vi "XGT 연속읽기 (독립)ONOFF.vi"() -> (1 "배열":i32[](array[numeric]))   [LabVIEW 2012]
uses:
  <vilib>/Instr/_visa.llb/VISA Configure Serial Port (Instr).vi
panel:
  in  "length":i32=6
  out "데이터 개수":string
  out "에러 코드":string
  out "Waveform Graph":i32[](graph)
  out "Array":i32[](array[numeric])
  out "Serial Settings:Number of Bytes at Serial Port":u32
  in  "stop bits (10: 1 bit)":u16(ring)=10 caption="정지 비트(10: 1비트)" items=["1.0"=10, "1.5"=15, "2.0"=20]
  in  "parity (0:none)":enum16{"None", "Odd", "Even", "Mark", "Space"}(ring) caption="패리티(0:없음)"
  in  "data bits (8)":u16=8 caption="데이터 비트(8)" min=5 max=8 step=1
  in  "baud rate (9600)":u32=9600 caption="보 전송속도(9600)"
  in  "VISA resource name":refnum<visa-resource-name>="COM4" caption="VISA 리소스 이름"
  # "응답"
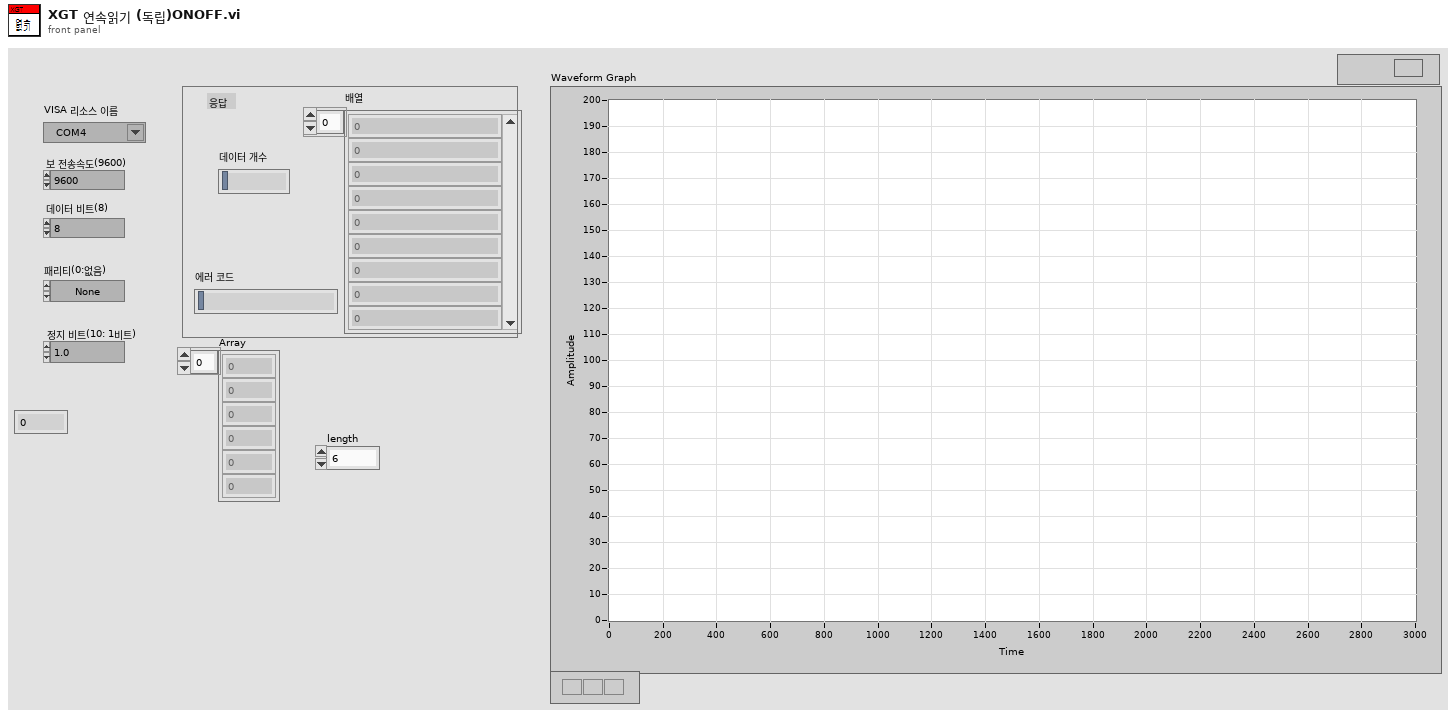
[diagram p1: front panel]
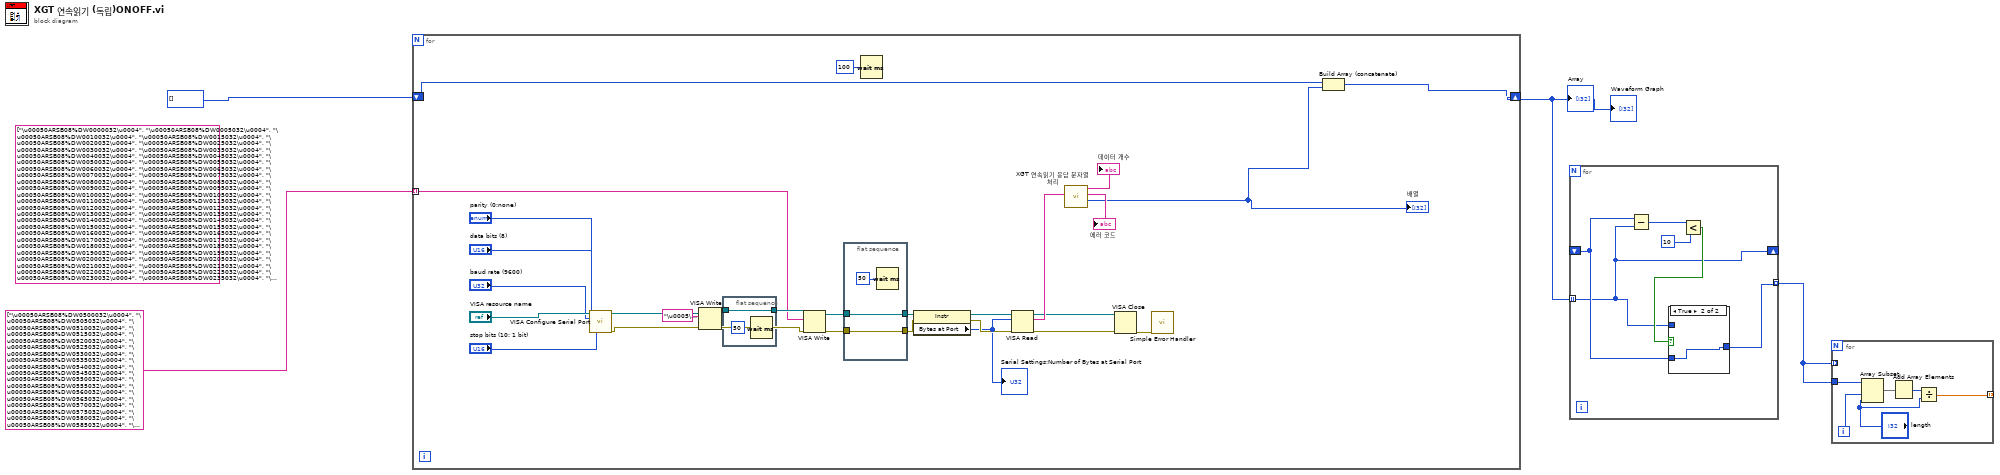
[diagram p0: block diagram]
diagram:
  (unwired) string[] ["\u00050ARSB08%DW0000032\u0004", "\u00050ARSB08%DW0005032\u0004", "\u00050ARSB08%DW0010032\u0004", "\u00050ARSB08%DW0015032\u0004", "\u00050ARSB08%DW0020032\u0004", "\u00050ARSB08%DW0025032\u0004", "\u00050ARSB08%DW0030032\u0004", "\u00050ARSB08%DW0035032\u0004", "\u00050ARSB08%DW0040032\u0004", "\u00050ARSB08%DW0045032\u0004", "\u00050ARSB08%DW0050032\u0004", "\u00050ARSB08%DW0055032\u0004", "\u00050ARSB08%DW0060032\u0004", "\u00050ARSB08%DW0065032\u0004", "\u00050ARSB08%DW0070032\u0004", "\u00050ARSB08%DW0075032\u0004", "\u00050ARSB08%DW0080032\u0004", "\u00050ARSB08%DW0085032\u0004", "\u00050ARSB08%DW0090032\u0004", "\u00050ARSB08%DW0095032\u0004", "\u00050ARSB08%DW0100032\u0004", "\u00050ARSB08%DW0105032\u0004", "\u00050ARSB08%DW0110032\u0004", "\u00050ARSB08%DW0115032\u0004", "\u00050ARSB08%DW0120032\u0004", "\u00050ARSB08%DW0125032\u0004", "\u00050ARSB08%DW0130032\u0004", "\u00050ARSB08%DW0135032\u0004", "\u00050ARSB08%DW0140032\u0004", "\u00050ARSB08%DW0145032\u0004", "\u00050ARSB08%DW0150032\u0004", "\u00050ARSB08%DW0155032\u0004", "\u00050ARSB08%DW0160032\u0004", "\u00050ARSB08%DW0165032\u0004", "\u00050ARSB08%DW0170032\u0004", "\u00050ARSB08%DW0175032\u0004", "\u00050ARSB08%DW0180032\u0004", "\u00050ARSB08%DW0185032\u0004", "\u00050ARSB08%DW0190032\u0004", "\u00050ARSB08%DW0195032\u0004", "\u00050ARSB08%DW0200032\u0004", "\u00050ARSB08%DW0205032\u0004", "\u00050ARSB08%DW0210032\u0004", "\u00050ARSB08%DW0215032\u0004", "\u00050ARSB08%DW0220032\u0004", "\u00050ARSB08%DW0225032\u0004", "\u00050ARSB08%DW0230032\u0004", "\u00050ARSB08%DW0235032\u0004", "\u00050ARSB08%DW0240032\u0004", "\u00050ARSB08%DW0245032\u0004", "\u00050ARSB08%DW0250032\u0004", "\u00050ARSB08%DW0255032\u0004", "\u00050ARSB08%DW0260032\u0004", "\u00050ARSB08%DW0265032\u0004", "\u00050ARSB08%DW0270032\u0004", "\u00050ARSB08%DW0275032\u0004", "\u00050ARSB08%DW0280032\u0004", "\u00050ARSB08%DW0285032\u0004", "\u00050ARSB08%DW0290032\u0004", "\u00050ARSB08%DW0295032\u0004"] ("Array")
  n1 = for {
    tunnel: string[] ["\u00050ARSB08%DW0500032\u0004", "\u00050ARSB08%DW0505032\u0004", "\u00050ARSB08%DW0510032\u0004", "\u00050ARSB08%DW0515032\u0004", "\u00050ARSB08%DW0520032\u0004", "\u00050ARSB08%DW0525032\u0004", "\u00050ARSB08%DW0530032\u0004", "\u00050ARSB08%DW0535032\u0004", "\u00050ARSB08%DW0540032\u0004", "\u00050ARSB08%DW0545032\u0004", "\u00050ARSB08%DW0550032\u0004", "\u00050ARSB08%DW0555032\u0004", "\u00050ARSB08%DW0560032\u0004", "\u00050ARSB08%DW0565032\u0004", "\u00050ARSB08%DW0570032\u0004", "\u00050ARSB08%DW0575032\u0004", "\u00050ARSB08%DW0580032\u0004", "\u00050ARSB08%DW0585032\u0004", "\u00050ARSB08%DW0590032\u0004", "\u00050ARSB08%DW0595032\u0004", "\u00050ARSB08%DW0600032\u0004", "\u00050ARSB08%DW0605032\u0004", "\u00050ARSB08%DW0610032\u0004", "\u00050ARSB08%DW0615032\u0004", "\u00050ARSB08%DW0620032\u0004", "\u00050ARSB08%DW0625032\u0004", "\u00050ARSB08%DW0630032\u0004", "\u00050ARSB08%DW0635032\u0004", "\u00050ARSB08%DW0640032\u0004", "\u00050ARSB08%DW0645032\u0004", "\u00050ARSB08%DW0650032\u0004", "\u00050ARSB08%DW0655032\u0004", "\u00050ARSB08%DW0660032\u0004", "\u00050ARSB08%DW0665032\u0004", "\u00050ARSB08%DW0670032\u0004", "\u00050ARSB08%DW0675032\u0004", "\u00050ARSB08%DW0680032\u0004", "\u00050ARSB08%DW0685032\u0004", "\u00050ARSB08%DW0690032\u0004", "\u00050ARSB08%DW0695032\u0004", "\u00050ARSB08%DW0700032\u0004", "\u00050ARSB08%DW0705032\u0004", "\u00050ARSB08%DW0710032\u0004", "\u00050ARSB08%DW0715032\u0004", "\u00050ARSB08%DW0720032\u0004", "\u00050ARSB08%DW0725032\u0004", "\u00050ARSB08%DW0730032\u0004", "\u00050ARSB08%DW0735032\u0004", "\u00050ARSB08%DW0740032\u0004", "\u00050ARSB08%DW0745032\u0004", "\u00050ARSB08%DW0750032\u0004", "\u00050ARSB08%DW0755032\u0004", "\u00050ARSB08%DW0760032\u0004", "\u00050ARSB08%DW0765032\u0004", "\u00050ARSB08%DW0770032\u0004", "\u00050ARSB08%DW0775032\u0004", "\u00050ARSB08%DW0780032\u0004", "\u00050ARSB08%DW0785032\u0004", "\u00050ARSB08%DW0790032\u0004", "\u00050ARSB08%DW0795032\u0004"] ("Array") -> [w8] mode=indexing
    shift-right: [w6] -> w1
    shift-left: i32[] [] -> [w5]
    n2 = call-poly "VISA Configure Serial Port"("VISA resource name"="VISA resource name", "baud rate (9600)"="baud rate (9600)", "data bits (8)"="data bits (8)", "parity (0:none)"="parity (0:none)", "stop bits (10: 1 bit)"="stop bits (10: 1 bit)") -> ("VISA resource name out"=w17:refnum<visa-resource-name>, "error out"=w16:errorcluster)  [unwired: 9 in]
    n3 = VISA Write(VISA resource name=w17, write buffer="\u0005\u0004", error in (no error)=w16) -> (VISA resource name out=w14:refnum<visa-resource-name>, error out=w15:errorcluster)  [unwired: 1 out]
    n4 = flat-sequence {
      tunnel: w14 -> [w35]
      tunnel: [w35] -> w13
      frame #0 {
        n5 = Wait (ms)(milliseconds to wait=u32 50) -> ()  [unwired: 1 out]
      }
    }
    n6 = VISA Write(VISA resource name=w13, write buffer=w8, error in (no error)=w15) -> (VISA resource name out=w32:refnum<visa-resource-name>, error out=w33:errorcluster)  [unwired: 1 out]
    n7 = flat-sequence {
      tunnel: w33 -> [w38]
      tunnel: [w38] -> w29
      tunnel: w32 -> [w37]
      tunnel: [w37] -> w30
      frame #0 {
        n8 = Wait (ms)(milliseconds to wait=u32 50 ("대기 시간(ms)")) -> ()  [unwired: 1 out]
      }
    }
    n9 = Wait (ms)(milliseconds to wait=u32 100 ("대기 시간(ms)")) -> ()  [unwired: 1 out]
    n10 = property class="Instr"(reference=w30, error in=w29) -> (reference out=w28:refnum<visa-resource-name>, error out=w31:errorcluster, "Bytes at Port"=w27:u32)
    "Serial Settings:Number of Bytes at Serial Port" <- w27
    n11 = VISA Read(VISA resource name=w28, byte count=w27, error in (no error)=w31) -> (VISA resource name out=w25:refnum<visa-resource-name>, read buffer=w26:string, error out=w18:errorcluster)  [unwired: 1 out]
    n12 = call "XGT 연속읽기 응답 문자열 처리.vi"("응답"=w26) -> ("배열"=w7:i32[], "에러 코드"=→"에러 코드":string, "데이터 개수"=→"데이터 개수":string)  [unwired: 5 in, 3 out]
    "배열" <- w7
    n13 = VISA Close(VISA resource name=w25, error in (no error)=w18) -> (error out=w24:errorcluster)
    n14 = call <vilib>:"Simple Error Handler.vi"("error in (no error)"=w24) -> ()  [unwired: 4 in, 5 out]
    n15 = Build Array (concatenate)(w5, w7) -> (w6:i32[])
  }
  "Array" <- w1
  "Waveform Graph" <- w1
  n16 = for {
    tunnel: w1 -> [w40] mode=indexing
    tunnel: [w44] -> w3 mode=indexing
    shift-right: [w40] -> _
    shift-left: _ -> [w43]
    n17 = Subtract(x=w43, y=w40) -> (x-y=w39:i32)
    n18 = Less?(x=w39, y=10) -> (x < y?=w41:bool)
    n19 = case shown="True" w41 {
      tunnel: w40 -> [w45 _]
      tunnel: w43 -> [_ w46]
      tunnel: [w45 w46] -> w44
      frame False {
      }
      frame True {
      }
    }
  }
  n20 = for {
    tunnel: w3 -> [w52]
    tunnel: [w47] -> _ mode=indexing
    tunnel: w3 -> [_] mode=indexing
    i -> [w51]
    n21 = Array Subset(array=w52, index=w51, length="length") -> (w50:i32[])
    n22 = Add Array Elements(numeric array=w50) -> (sum=w49:i32)
    n23 = Divide(x=w49, y="length") -> (x/y=w47:dbl)
  }
